vi "Data Processor.vi"(8 "error in (no error)":errorcluster) -> (0 "error out":errorcluster)   [LabVIEW 2014]
doc: "This VI runs at startup of the AddressBook web service. It manages the lifetime of the address book data store by loading the data at start and saving the data periodically and at web service shutdown."
uses:
  <vilib>/Utility/sysdir.llb/System Directory Type.ctl
  Libraries/Contact Data/Contact Data.lvlib
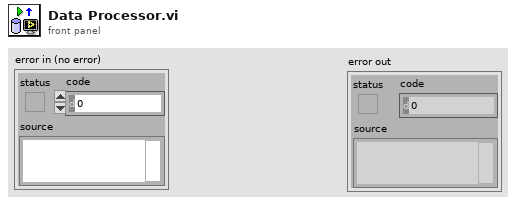
[diagram p1: front panel]
types:
  T1 = typedef "System Directory Type.ctl" = i32
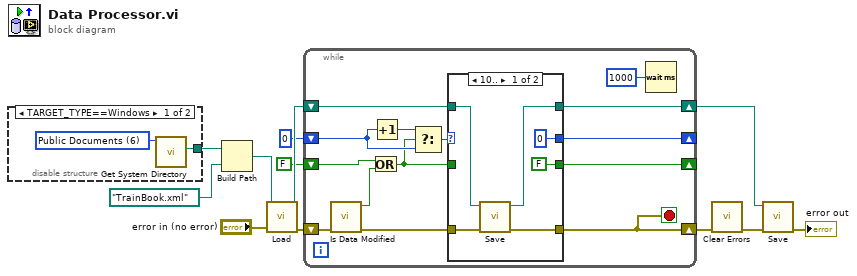
[diagram p0: block diagram]
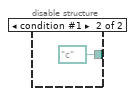
[diagram p2: hidden frame]
diagram:
  n1 = disable-structure shown="TARGET_TYPE==Windows" {
    disable-tunnel: [w13 path "c:/" ("system directory")] -> w6
    frame condition #0 (active) {
      w14 = T1 6 items=["User Home"=0, "User Desktop"=1, "User Documents"=2, "User Application Data"=3, "User Preferences"=4, "User Temporary"=5, "Public Documents"=6, "Public Application Data"=7, "Public Preferences"=8, "Public Cache"=13, "System Core Libraries"=9, "System Installed Libraries"=10, "Application Files"=11, "Boot Volume Root"=12] ("system directory type")
      n2 = call <vilib>:"Get System Directory.vi"("system directory type"=w14) -> ("system directory"=w13:path)  [unwired: 10 in]
    }
    frame condition #1 {
    }
  }
  n3 = Build Path(base path=w6, name or relative path=path "TrainBook.xml") -> (appended path=w4:path)
  n4 = call "Load.vi"("error in (no error)"="error in (no error)", "Data File"=w4) -> ("error out"=w12:errorcluster, "dup Data File"=w10:path)  [unwired: 8 in]
  n5 = while {
    shift-right: [w16] -> w11
    shift-left: w12 -> [w28]
    shift-right: [w18] -> w9
    shift-left: w10 -> [w19]
    shift-right: [w22] -> _
    shift-left: 0 -> [w25]
    shift-right: [w20] -> _
    shift-left: FALSE -> [w27]
    stop <- w16 stop-if-true
    n6 = call "Is Data Modified.vi"("error in (no error)"=w28) -> ("error out"=w17:errorcluster, "Data Modified?"=w26:bool)  [unwired: 9 in]
    n7 = Or(x=w27, y=w26) -> (x .or. y?=w21:bool)
    n8 = Increment(x=w25) -> (x+1=w24:i32)
    n9 = Select(t=w24, s=w21, f=w25) -> (s? t:f=w23:i32)
    n10 = case shown="10.." w23 {
      selector: w23 -> [_ w39]
      tunnel: [0 w39] -> w22
      tunnel: w21 -> [_ w38]
      tunnel: [FALSE w38] -> w20
      tunnel: w19 -> [w35 w37]
      tunnel: [w34 w37] -> w18
      tunnel: [w31 w36] -> w16
      tunnel: w17 -> [w30 w36]
      frame 10.. {
        n11 = call "Save.vi"("error in (no error)"=w30, "Data File"=w35) -> ("error out"=w31:errorcluster, "dup Data File"=w34:path)  [unwired: 8 in]
      }
      frame Default {
      }
    }
    n12 = Wait (ms)(milliseconds to wait=u32 1000) -> ()  [unwired: 1 out]
  }
  n13 = call <vilib>:"Clear Errors.vi"("error in (no error)"=w11) -> ("error out"=w3:errorcluster)  [unwired: 5 in, 1 out]
  n14 = call "Save.vi"("error in (no error)"=w3, "Data File"=w9) -> ("error out"=→"error out":errorcluster)  [unwired: 8 in, 1 out]
